vi "Encoder_Config_Simulation_Global.vi"(0 "EncoderIndex":T2, 5 "menu":enum16{"set", "get", "delete"}(ring)=enum."get", 7 "Encoder Config set":T1, 11 "error in (no error)":errorcluster) -> (8 "Encoder Config get":T1, 15 "error out":errorcluster)   [LabVIEW 2017]
uses:
  <vilib>/Rock Robotics/SystemInterfaces/Encoder/FPGA_EncoderIdx.ctl
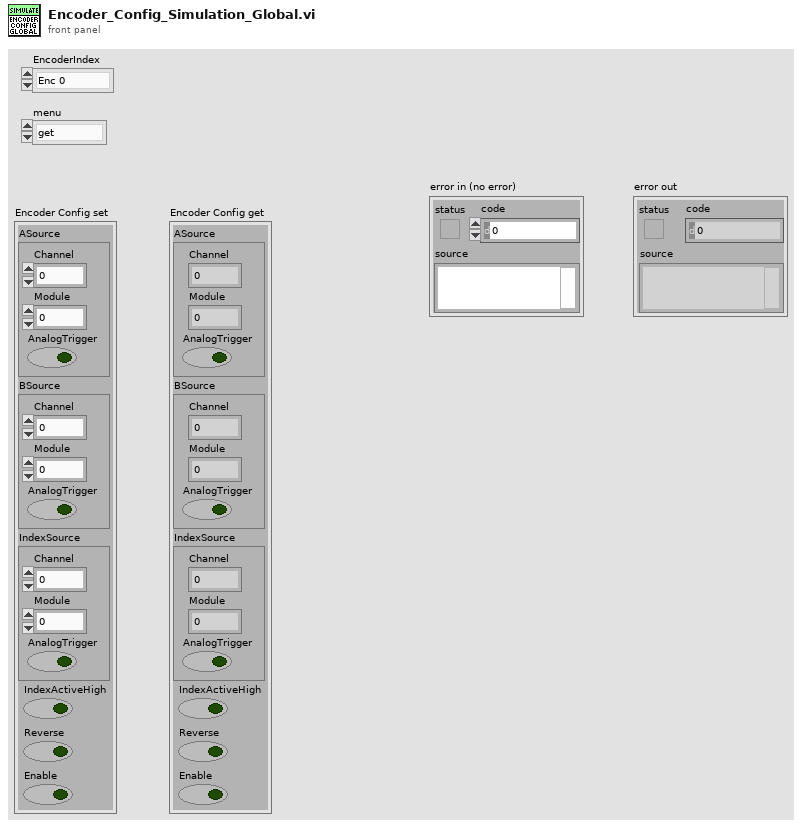
[diagram p1: front panel]
types:
  T1 = cluster{"ASource":cluster{"Channel":fxp<+,4,4>, "Module":fxp<+,1,1>, "AnalogTrigger":bool}, "BSource":cluster{"Channel":fxp<+,4,4>, "Module":fxp<+,1,1>, "AnalogTrigger":bool}, "IndexSource":cluster{"Channel":fxp<+,4,4>, "Module":fxp<+,1,1>, "AnalogTrigger":bool}, "IndexActiveHigh":bool, "Reverse":bool, "Enable":bool}
  T2 = typedef "FPGA_EncoderIdx.ctl" = enum8{"Enc 0", "Enc 1", "Enc 2", "Enc 3", "Enc 4", "Enc 5", "Enc 6", "Enc 7", "Invalid"}
  T3 = cluster{"ASource":cluster{"Channel":fxp<+,4,4>, "Module":fxp<+,1,1>, "AnalogTrigger":bool}, "BSource":cluster{"Channel":fxp<+,4,4>, "Module":fxp<+,1,1>, "AnalogTrigger":bool}, "IndexSource":cluster{"Channel":fxp<+,4,4>, "Module":fxp<+,1,1>, "AnalogTrigger":bool}, "IndexActiveHigh":bool, "Reverse":bool, "Enable":bool}[]
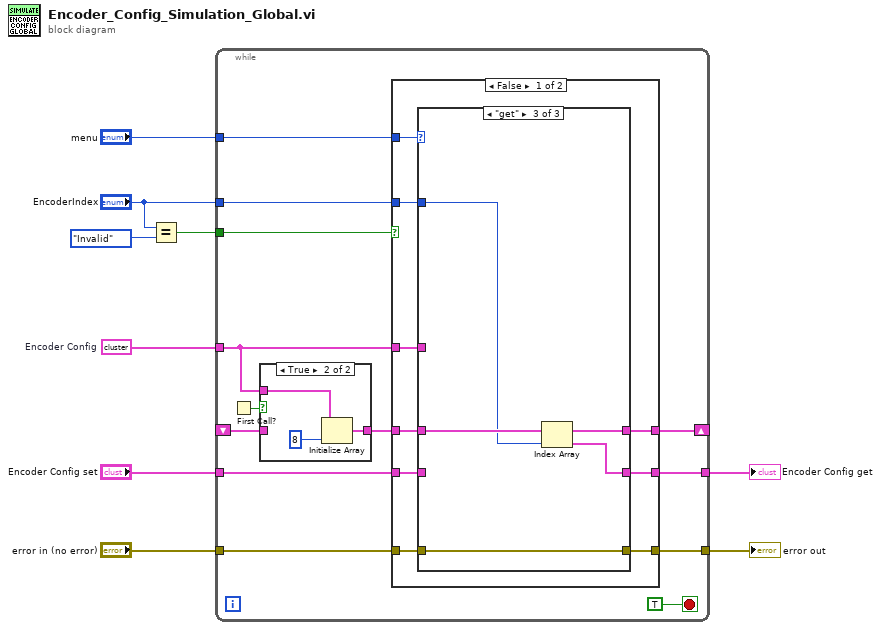
[diagram p0: block diagram]
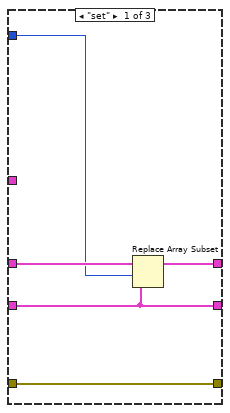
[diagram p2: hidden frame]
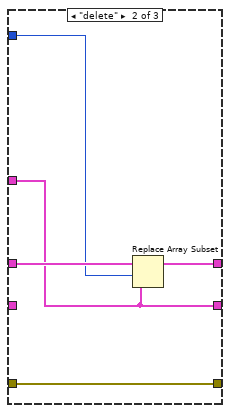
[diagram p3: hidden frame]
diagram:
  w1 = T1 {"ASource"={"Channel"=0.0, "Module"=0.0, "AnalogTrigger"=FALSE}, "BSource"={"Channel"=0.0, "Module"=0.0, "AnalogTrigger"=FALSE}, "IndexSource"={"Channel"=0.0, "Module"=0.0, "AnalogTrigger"=FALSE}, "IndexActiveHigh"=FALSE, "Reverse"=FALSE, "Enable"=FALSE}  # Encoder Config
  n1 = Equal?(x="EncoderIndex", y=FPGA_EncoderIdx."Invalid" ("EncoderIndex")) -> (x = y?=w7:bool)
  n2 = while {
    tunnel: "Encoder Config set" -> [w22]
    tunnel: "error in (no error)" -> [w18]
    shift-right: [w21] -> _
    shift-left: _ -> [w13]
    tunnel: [w20] -> w2
    tunnel: "menu" -> [w19]
    tunnel: [w17] -> w8
    tunnel: "EncoderIndex" -> [w12]
    tunnel: w7 -> [w11]
    tunnel: w1 -> [w10]
    stop <- TRUE stop-if-true
    n3 = First Call?() -> (First Call?: T/F=w15:bool)
    n4 = case shown="True" w15 {
      tunnel: [w49 w51] -> w14
      tunnel: w13 -> [w49 _]
      tunnel: w10 -> [_ w50]
      frame False {
      }
      frame True {
        n5 = Initialize Array(w50, 8 ("dimension size")) -> (w51:T3)
      }
    }
    n6 = case shown="False" w11 {
      tunnel: w22 -> [w31 _]
      tunnel: [w30 w48] -> w21
      tunnel: [w29 w46] -> w20
      tunnel: w19 -> [w28 _]
      tunnel: w18 -> [w27 w47]
      tunnel: [w26 w47] -> w17
      tunnel: w14 -> [w25 w48]
      tunnel: w12 -> [w24 _]
      tunnel: w10 -> [w23 w46]
      frame False {
        n7 = case shown="\"get\"" w28 {
          tunnel: w31 -> [w34 _ _]
          tunnel: [w35 w40 w45] -> w30
          tunnel: w25 -> [w36 w41 w45]
          tunnel: [w34 w37 w44] -> w29
          tunnel: [w33 w39 w43] -> w26
          tunnel: w27 -> [w33 w39 w43]
          tunnel: w24 -> [w32 w38 w42]
          tunnel: w23 -> [_ w37 _]
          frame "set" {
            n8 = Replace Array Subset(array=w36, new element=w34, index=w32) -> (w35:T3)
          }
          frame "delete" {
            n9 = Replace Array Subset(array=w41, new element=w37, index=w38) -> (w40:T3)
          }
          frame "get" {
            n10 = Index Array(array=w45, index=w42) -> (element=w44:T1)
          }
        }
      }
      frame True {
        # "Do nothing if Invalid."
      }
    }
  }
  "error out" <- w8
  "Encoder Config get" <- w2
